vi "UI Refresh Data.vi"(8 "error in (no error)":errorcluster, 11 "GObject View in":refnum<class "VI View.lvclass">) -> (0 "error out":errorcluster, 3 "GObject View out":refnum<class "VI View.lvclass">)   [LabVIEW 2013, in "SET Project Editor.lvlib" / "VI View.lvclass"]
uses:
  VI View.lvclass
  VI View.lvclass/VI View.ctl
  UI View/UI View.lvclass/UI View.ctl
  SET Project Data/Project Data Class/Project Data.lvclass
  SET Project Data/VI Class/VI Data.lvclass
  UI View/Read _LangData.vi
  UI View/Read UUID.vi
  SET Project Data/Control Classes/GObject/Read Label.vi
  SET Project Data/Control Classes/GObject/Read ClassName.vi
  SET Project Data/Control Classes/GObject/Read UID.vi
  SET Project Data/Control Classes/GObject/GObject.lvclass
  SET Project Editor.lvlib
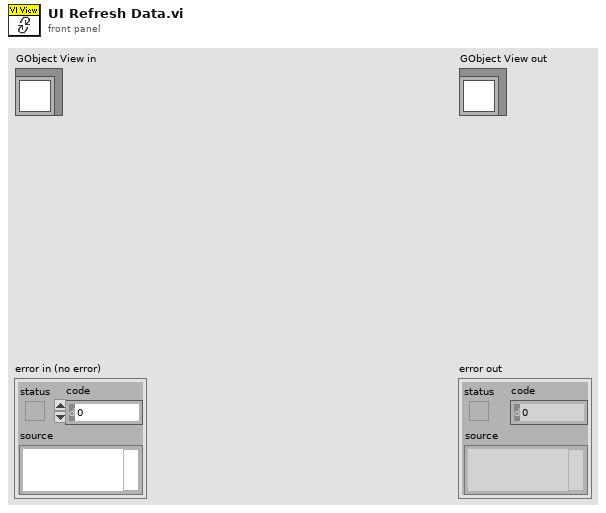
[diagram p1: front panel]
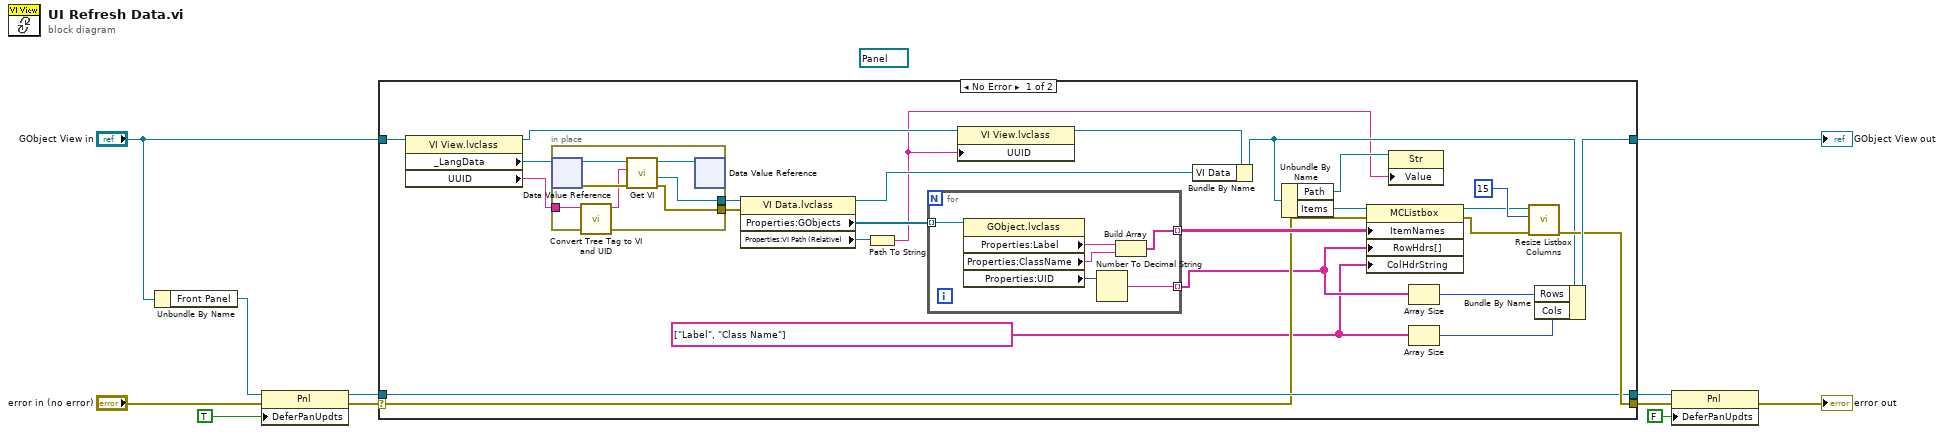
[diagram p0: block diagram]
diagram:
  (unwired) refnum<vi> refnum ("Front Panel")
  n1 = Unbundle By Name("GObject View in") -> ("Front Panel"=w9:refnum<vi>)
  n2 = property class="Pnl"(reference=w9, error in="error in (no error)", "DeferPanUpdts"=TRUE ("Defer Panel Updates")) -> (reference out=w5:refnum<vi>, error out=w6:errorcluster)
  n3 = case shown="No Error" w6 {
    selector: w6 -> [w26 w53]
    tunnel: [w32 w53] -> w3
    tunnel: [w36 w52] -> w11
    tunnel: "GObject View in" -> [w22 w52]
    tunnel: w5 -> [w29 w51]
    tunnel: [w29 w51] -> w4
    frame No Error {
      w24 = string[] ["Label", "Class Name"]
      n4 = property class="VI View.lvclass"(reference=w22) -> (reference out=w16:refnum<class "VI View.lvclass">, "_LangData"=w21:refnum<data-value>, "UUID"=w20:string)  [unwired: 1 in, 1 out]
      n5 = in-place {
        in-place-border: w20 -> [w41]
        in-place-border: [w39] -> w19
        in-place-border: [w38] -> w18
        n6 = in-place-dvr #1(w21) -> (w44:refnum<class "Project Data.lvclass">, w42:errorcluster)
        n7 = call "Convert Tree Tag to VI and UID.vi"("Tree Tag"=w41) -> ("File Path (Relative)"=w40:string)  [unwired: 7 in, 3 out]
        n8 = call-dynamic "Get VI.vi"("error in (no error)"=w42, "VI Path (Relative)"=w40, "ProjectData in"=w44) -> ("error out"=w38:errorcluster, "VI Data out"=w39:refnum<class "VI Data.lvclass">, "ProjectData out"=w43:refnum<class "Project Data.lvclass">)  [unwired: 5 in, 1 out]
        n9 = in-place-dvr #1(w43) -> ()  [unwired: 2 out]
      }
      n10 = property class="VI Data.lvclass"(reference=w19, error in=w18) -> (reference out=w17:refnum<class "VI Data.lvclass">, "Properties:GObjects"=w28:refnum<class "GObject.lvclass">[], "Properties:VI Path (Relative)"=w14:path)  [unwired: 1 out]
      n11 = Path To String(path=w14) -> (string=w12:string)
      n12 = for {
        tunnel: [w45] -> w37 mode=indexing
        tunnel: w28 -> [w50] mode=indexing
        tunnel: [w48] -> w25 mode=indexing
        n13 = property class="GObject.lvclass"(reference=w50) -> ("Properties:Label"=w47:string, "Properties:ClassName"=w46:string, "Properties:UID"=w49:i32)  [unwired: 1 in, 2 out]
        n14 = Number To Decimal String(number=w49) -> (decimal integer string=w48:string)  [unwired: 1 in]
        n15 = Build Array(w47, w46) -> (w45:string[])
      }
      n16 = property class="VI View.lvclass"(reference=w16, "UUID"=w12) -> (reference out=w15:refnum<class "VI View.lvclass">)  [unwired: 1 in, 1 out]
      n17 = Bundle By Name(cluster=w15, "VI Data"=w17) -> (w23:refnum<class "VI View.lvclass">)
      n18 = Unbundle By Name(w23) -> ("Path"=w13:refnum<vi>, "Items"=w27:refnum<vi>)
      n19 = property class="MCListbox"(reference=w27, error in=w26, "ItemNames"=w37, "RowHdrs[]"=w25, "ColHdrString"=w24) -> (reference out=w34:refnum<vi>, error out=w33:errorcluster)
      n20 = property class="Str"(reference=w13, "Value"=w12) -> ()  [unwired: 1 in, 2 out]
      n21 = Array Size(array=w25) -> (size(s)=w31:i32)
      n22 = Array Size(array=w24) -> (size(s)=w30:i32)
      n23 = call "Resize Listbox Columns.vi"("error in (no error)"=w33, "Padding (5px)"=i16 15, "Listbox Control ref in"=w34) -> ("error out"=w32:errorcluster)  [unwired: 7 in, 1 out]
      n24 = Bundle By Name(cluster=w23, "Rows"=w31, "Cols"=w30) -> (w36:refnum<class "VI View.lvclass">)
    }
    frame Error {
    }
  }
  "GObject View out" <- w11
  n25 = property class="Pnl"(reference=w4, error in=w3, "DeferPanUpdts"=FALSE ("Defer Panel Updates")) -> (error out=→"error out":errorcluster)  [unwired: 1 out]
